vi "rohitdecimal to binary.vi"() -> ()   [LabVIEW 2009]
panel:
  in  "Slide":dbl(slide) scale=0.0..7.0 scale format="%#.6g"
  out "fours":bool
  out "twos":bool
  out "ones":bool
  in  "stop":bool
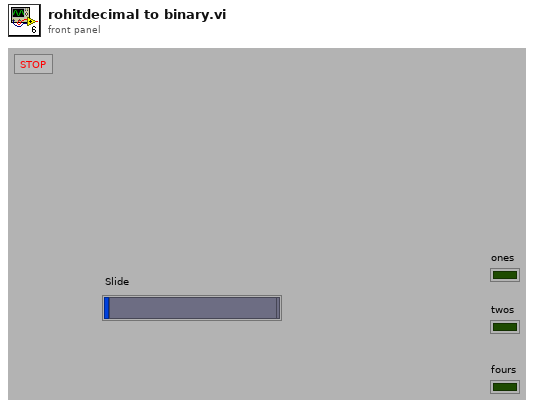
[diagram p1: front panel]
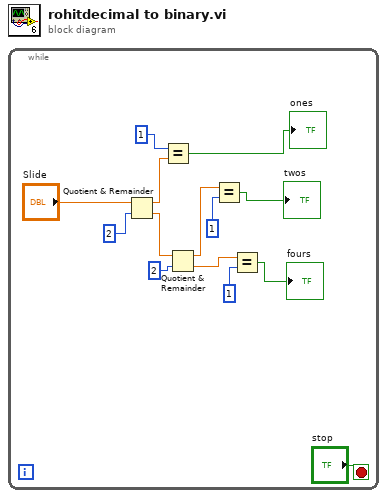
[diagram p0: block diagram]
diagram:
  n1 = while {
    stop <- "stop" stop-if-true
    n2 = Quotient & Remainder(x="Slide", y=2) -> (x-y*floor(x/y)=w12:dbl, floor(x/y)=w13:dbl)
    n3 = Equal?(x=1, y=w12) -> (x = y?=→"ones":bool)
    n4 = Quotient & Remainder(x=w13, y=2) -> (x-y*floor(x/y)=w10:dbl, floor(x/y)=w7:dbl)
    n5 = Equal?(x=w10, y=1) -> (x = y?=→"twos":bool)
    n6 = Equal?(x=w7, y=1) -> (x = y?=→"fours":bool)
  }
